vi "Set Switch State V2.vi"(5 "Action":T1(ring)=enum."Connect PulseGen to CH2", 7 "State":bool, 11 "error in (no error)":errorcluster) -> (15 "error out":errorcluster)   [LabVIEW 2010]
uses:
  <vilib>/DAQmx/write.llb/DAQmx Write (Digital 1D Bool 1Chan 1Samp).vi
  <vilib>/DAQmx/write.llb/DAQmx Write (Digital U8 1Chan 1Samp).vi
  <vilib>/DAQmx/create/channels.llb/DAQmx Create Channel (DO-Digital Output).vi
  <vilib>/daqmx/miscellaneous.llb/DAQmx Fill In Error Info.vi
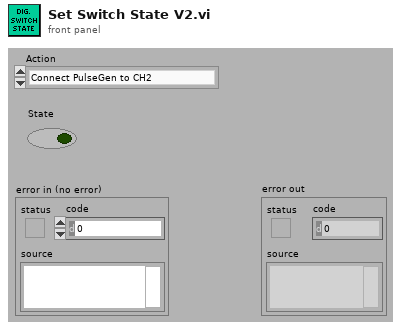
[diagram p1: front panel]
types:
  T1 = enum16{"--Disconnect All--", "Connect PulseGen to CH1", "Connect PulseGen to CH2", "Connect PulseGen to CH3", "Connect PulseGen to CH4", "Connect PulseGen to CH5", "Connect PulseGen to CH6", "Connect PulseGen to CH7", "Connect PulseGen to CH8", "Connect PulseGen to CH9", "Connect PulseGen to CH10", "Connect PulseGen to CH11", "Connect PulseGen to CH12", "Connect PulseGen to CH13", "Connect PulseGen to CH14", "Connect PulseGen to CH15", "Connect PulseGen to CH16", "Connect PulseGen to CH17", "Connect PulseGen to CH18", "Connect PulseGen to CH19", "Connect PulseGen to CH20", "Connect PulseGen to CH21", "Connect PulseGen to CH22", "Connect PulseGen to CH23", "Connect PulseGen to CH24", "Connect PulseGen to CH25", "Set MAG_SW", "Set Dynamic Load", "Set Expansion Trigger", "Trigger Positive Pulse", "Trigger Negative Pulse", "Set MSP Magic Pin", "Set BAT_EN", "Connect MSP_ACLK to CTR", "Connect MSP_MCLK to CTR", "Connect MSP_DIG_TST_OUT to CTR", "Connect STIM_SCK to CTR", "Connect STIM_CLK to CTR", "Connect SMU2 to Magnet", "Magnet Enable", "Cap Short", "Connect Positive Pulse to Pulse Bus", "Connect Negative Pulse to Pulse Bus", "Connect JTAG", "Connect JTAG DVDD Power", "RF Attach", "Connect SMU3 to VBAT", "Connect SMU3 Soft Start", "Connect ARB to Charge Coil", "Connect ARB to Matrix", "Connect CTR to Matrix", "DMM_I Short", "DMM_I 1000 Ohm", "DMM_I 100 Ohm", "DMM_I 10 Ohm", "Connect CH25 to DUT GND", "Enclosure Lights", "Heat Fan Zone 1", "Heat Fan Zone 2", "Temp Zone 1", "Temp Zone 2", "Temp Zone 3", "Guard Door Locks", "Air Heat Zone 3", "Zone 3 Vent", "Zone 3 Loader", "Zone 3 Upper Bed", "Zone 3 Lower Bed", "Zone 3 Standby Temp", "Yellow Light", "Red Light", "Green Light", "Reset Common Test Lines"}
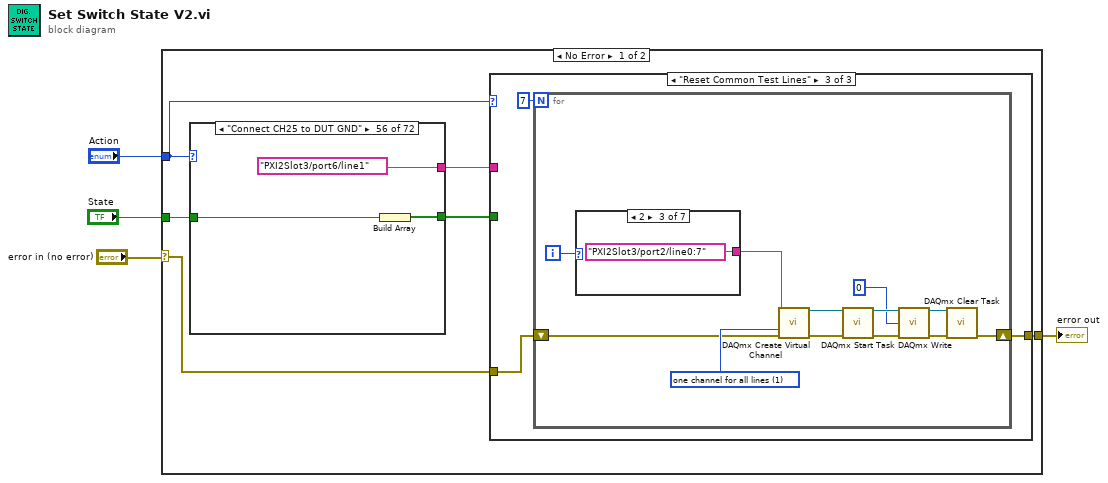
[diagram p0: block diagram]
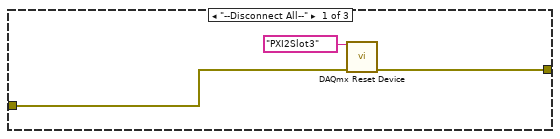
[diagram p2: hidden frame]
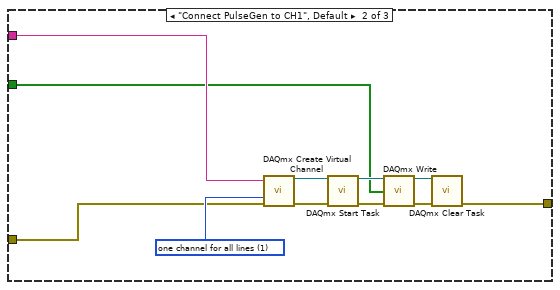
[diagram p3: hidden frame]
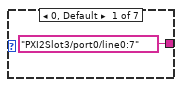
[diagram p4: hidden frame]
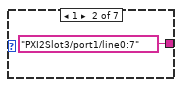
[diagram p5: hidden frame]
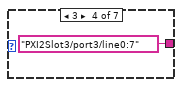
[diagram p6: hidden frame]
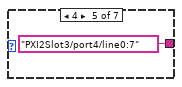
[diagram p7: hidden frame]
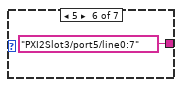
[diagram p8: hidden frame]
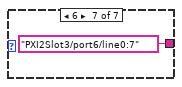
[diagram p9: hidden frame]
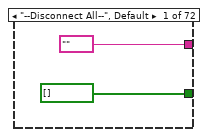
[diagram p10: hidden frame]
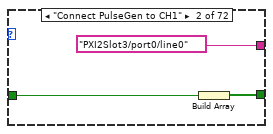
[diagram p11: hidden frame]
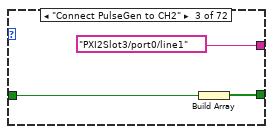
[diagram p12: hidden frame]
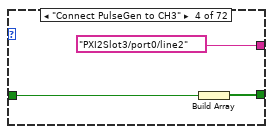
[diagram p13: hidden frame]
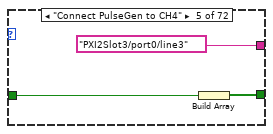
[diagram p14: hidden frame]
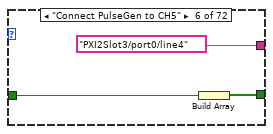
[diagram p15: hidden frame]
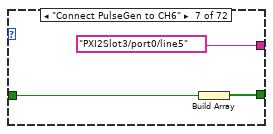
[diagram p16: hidden frame]
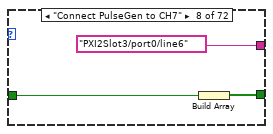
[diagram p17: hidden frame]
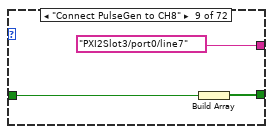
[diagram p18: hidden frame]
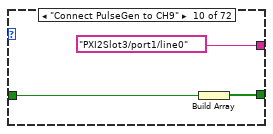
[diagram p19: hidden frame]
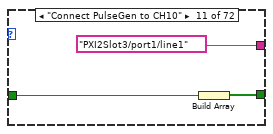
[diagram p20: hidden frame]
diagram:
  n1 = case shown="No Error" "error in (no error)" {
    selector: "error in (no error)" -> [w5 w263]
    tunnel: "State" -> [w8 _]
    tunnel: [w7 w263] -> w3
    tunnel: "Action" -> [w6 _]
    frame No Error {
      n2 = case shown="\"Connect CH25 to DUT GND\"" w6 {
        tunnel: [tag "" ("Lines") tag "PXI2Slot3/port0/line0" ("Lines") tag "PXI2Slot3/port0/line1" ("Lines") tag "PXI2Slot3/port0/line2" ("Lines") tag "PXI2Slot3/port0/line3" ("Lines") tag "PXI2Slot3/port0/line4" ("Lines") tag "PXI2Slot3/port0/line5" ("Lines") tag "PXI2Slot3/port0/line6" ("Lines") tag "PXI2Slot3/port0/line7" ("Lines") tag "PXI2Slot3/port1/line0" ("Lines") tag "PXI2Slot3/port1/line1" ("Lines") tag "PXI2Slot3/port1/line2" ("Lines") tag "PXI2Slot3/port1/line3" ("Lines") tag "PXI2Slot3/port1/line4" ("Lines") tag "PXI2Slot3/port1/line5" ("Lines") tag "PXI2Slot3/port1/line6" ("Lines") tag "PXI2Slot3/port1/line7" ("Lines") tag "PXI2Slot3/port2/line0" ("Lines") tag "PXI2Slot3/port2/line1" ("Lines") tag "PXI2Slot3/port2/line2" ("Lines") tag "PXI2Slot3/port2/line3" ("Lines") tag "PXI2Slot3/port2/line4" ("Lines") tag "PXI2Slot3/port2/line5" ("Lines") tag "PXI2Slot3/port2/line6" ("Lines") tag "PXI2Slot3/port2/line7" ("Lines") tag "PXI2Slot3/port3/line0" ("Lines") tag "PXI2Slot3/port3/line1" ("Lines") tag "PXI2Slot3/port3/line2:3" ("Lines") tag "PXI2Slot3/port3/line3" ("Lines") tag "PXI2Slot3/port3/line3:4" ("Lines") tag "PXI2Slot3/port3/line3:5" ("Lines") tag "PXI2Slot3/port3/line6" ("Lines") tag "PXI2Slot3/port3/line7" ("Lines") tag "PXI2Slot3/port4/line0" ("Lines") tag "PXI2Slot3/port4/line1" ("Lines") tag "PXI2Slot3/port4/line2" ("Lines") tag "PXI2Slot3/port4/line3" ("Lines") tag "PXI2Slot3/port4/line4" ("Lines") tag "PXI2Slot3/port4/line5" ("Lines") tag "PXI2Slot3/port4/line6" ("Lines") tag "PXI2Slot3/port4/line7" ("Lines") tag "PXI2Slot3/port5/line0" ("Lines") tag "PXI2Slot3/port5/line1" ("Lines") tag "PXI2Slot3/port5/line2" ("Lines") tag "PXI2Slot3/port5/line3" ("Lines") tag "PXI2Slot3/port5/line4" ("Lines") tag "PXI2Slot3/port5/line5" ("Lines") tag "PXI2Slot3/port5/line6" ("Lines") tag "PXI2Slot3/port5/line7" ("Lines") tag "PXI2Slot3/port6/line7" ("Lines") tag "PXI2Slot3/port6/line6" ("Lines") tag "PXI2Slot3/port6/line5" ("Lines") tag "PXI2Slot3/port6/line4" ("Lines") tag "PXI2Slot3/port6/line3" ("Lines") tag "PXI2Slot3/port6/line2" ("Lines") tag "PXI2Slot3/port6/line1" ("Lines") tag "PXI2Slot3/port8/line0" ("Lines") tag "PXI2Slot3/port8/line1" ("Lines") tag "PXI2Slot3/port8/line2" ("Lines") tag "PXI2Slot3/port8/line3" ("Lines") tag "PXI2Slot3/port8/line4" ("Lines") tag "PXI2Slot3/port8/line5" ("Lines") tag "PXI2Slot3/port8/line6" ("Lines") tag "PXI2Slot3/port8/line7" ("Lines") tag "PXI2Slot3/port9/line0" ("Lines") tag "PXI2Slot3/port9/line1" ("Lines") tag "PXI2Slot3/port9/line2" ("Lines") tag "PXI2Slot3/port9/line3" ("Lines") tag "PXI2Slot3/port9/line4" ("Lines") tag "PXI2Slot3/port9/line5" ("Lines") tag "PXI2Slot3/port9/line6" ("Lines") tag "PXI2Slot3/port9/line7" ("Lines")] -> w10
        tunnel: [bool[] [] w50 w53 w56 w59 w62 w65 w68 w71 w74 w77 w80 w83 w86 w89 w92 w95 w98 w101 w104 w107 w110 w113 w116 w119 w122 w125 w128 w131 w134 w138 w141 w144 w147 w150 w153 w156 w159 w162 w165 w168 w171 w174 w177 w180 w183 w186 w189 w192 w195 w198 w201 w204 w207 w210 w213 w216 w219 w222 w226 w229 w231 w234 w237 w240 w244 w246 w249 w252 w255 w258 w261] -> w9
        tunnel: w8 -> [_ w49 w52 w55 w58 w61 w64 w67 w70 w73 w76 w79 w82 w85 w88 w91 w94 w97 w100 w103 w106 w109 w112 w115 w118 w121 w124 w127 w130 w133 w137 w140 w143 w146 w149 w152 w155 w158 w161 w164 w167 w170 w173 w176 w179 w182 w185 w188 w191 w194 w197 w200 w203 w206 w209 w212 w215 w218 w221 w225 w228 w230 w233 w236 w239 w243 w245 w248 w251 w254 w257 w260]
        frame "--Disconnect All--", Default {
        }
        frame "Connect PulseGen to CH1" {
          n3 = Build Array(w49) -> (w50:bool[])
        }
        frame "Connect PulseGen to CH2" {
          n4 = Build Array(w52) -> (w53:bool[])
        }
        frame "Connect PulseGen to CH3" {
          n5 = Build Array(w55) -> (w56:bool[])
        }
        frame "Connect PulseGen to CH4" {
          n6 = Build Array(w58) -> (w59:bool[])
        }
        frame "Connect PulseGen to CH5" {
          n7 = Build Array(w61) -> (w62:bool[])
        }
        frame "Connect PulseGen to CH6" {
          n8 = Build Array(w64) -> (w65:bool[])
        }
        frame "Connect PulseGen to CH7" {
          n9 = Build Array(w67) -> (w68:bool[])
        }
        frame "Connect PulseGen to CH8" {
          n10 = Build Array(w70) -> (w71:bool[])
        }
        frame "Connect PulseGen to CH9" {
          n11 = Build Array(w73) -> (w74:bool[])
        }
        frame "Connect PulseGen to CH10" {
          n12 = Build Array(w76) -> (w77:bool[])
        }
        frame "Connect PulseGen to CH11" {
          n13 = Build Array(w79) -> (w80:bool[])
        }
        frame "Connect PulseGen to CH12" {
          n14 = Build Array(w82) -> (w83:bool[])
        }
        frame "Connect PulseGen to CH13" {
          n15 = Build Array(w85) -> (w86:bool[])
        }
        frame "Connect PulseGen to CH14" {
          n16 = Build Array(w88) -> (w89:bool[])
        }
        frame "Connect PulseGen to CH15" {
          n17 = Build Array(w91) -> (w92:bool[])
        }
        frame "Connect PulseGen to CH16" {
          n18 = Build Array(w94) -> (w95:bool[])
        }
        frame "Connect PulseGen to CH17" {
          n19 = Build Array(w97) -> (w98:bool[])
        }
        frame "Connect PulseGen to CH18" {
          n20 = Build Array(w100) -> (w101:bool[])
        }
        frame "Connect PulseGen to CH19" {
          n21 = Build Array(w103) -> (w104:bool[])
        }
        frame "Connect PulseGen to CH20" {
          n22 = Build Array(w106) -> (w107:bool[])
        }
        frame "Connect PulseGen to CH21" {
          n23 = Build Array(w109) -> (w110:bool[])
        }
        frame "Connect PulseGen to CH22" {
          n24 = Build Array(w112) -> (w113:bool[])
        }
        frame "Connect PulseGen to CH23" {
          n25 = Build Array(w115) -> (w116:bool[])
        }
        frame "Connect PulseGen to CH24" {
          n26 = Build Array(w118) -> (w119:bool[])
        }
        frame "Connect PulseGen to CH25" {
          n27 = Build Array(w121) -> (w122:bool[])
        }
        frame "Set MAG_SW" {
          n28 = Build Array(w124) -> (w125:bool[])
        }
        frame "Set Dynamic Load" {
          n29 = Build Array(w127, w127) -> (w128:bool[])
        }
        frame "Set Expansion Trigger" {
          n30 = Build Array(w130) -> (w131:bool[])
        }
        frame "Trigger Positive Pulse" {
          n31 = Build Array(w133, w133) -> (w134:bool[])
        }
        frame "Trigger Negative Pulse" {
          n32 = Build Array(w137, FALSE ("element"), w137) -> (w138:bool[])
        }
        frame "Set MSP Magic Pin" {
          n33 = Build Array(w140) -> (w141:bool[])
        }
        frame "Set BAT_EN" {
          n34 = Build Array(w143) -> (w144:bool[])
        }
        frame "Connect MSP_ACLK to CTR" {
          n35 = Build Array(w146) -> (w147:bool[])
        }
        frame "Connect MSP_MCLK to CTR" {
          n36 = Build Array(w149) -> (w150:bool[])
        }
        frame "Connect MSP_DIG_TST_OUT to CTR" {
          n37 = Build Array(w152) -> (w153:bool[])
        }
        frame "Connect STIM_SCK to CTR" {
          n38 = Build Array(w155) -> (w156:bool[])
        }
        frame "Connect STIM_CLK to CTR" {
          n39 = Build Array(w158) -> (w159:bool[])
        }
        frame "Connect SMU2 to Magnet" {
          n40 = Build Array(w161) -> (w162:bool[])
        }
        frame "Magnet Enable" {
          n41 = Build Array(w164) -> (w165:bool[])
        }
        frame "Cap Short" {
          n42 = Build Array(w167) -> (w168:bool[])
        }
        frame "Connect Positive Pulse to Pulse Bus" {
          n43 = Build Array(w170) -> (w171:bool[])
        }
        frame "Connect Negative Pulse to Pulse Bus" {
          n44 = Build Array(w173) -> (w174:bool[])
        }
        frame "Connect JTAG" {
          n45 = Build Array(w176) -> (w177:bool[])
        }
        frame "Connect JTAG DVDD Power" {
          n46 = Build Array(w179) -> (w180:bool[])
        }
        frame "RF Attach" {
          n47 = Build Array(w182) -> (w183:bool[])
        }
        frame "Connect SMU3 to VBAT" {
          n48 = Build Array(w185) -> (w186:bool[])
        }
        frame "Connect SMU3 Soft Start" {
          n49 = Build Array(w188) -> (w189:bool[])
        }
        frame "Connect ARB to Charge Coil" {
          n50 = Build Array(w191) -> (w192:bool[])
        }
        frame "Connect ARB to Matrix" {
          n51 = Build Array(w194) -> (w195:bool[])
        }
        frame "Connect CTR to Matrix" {
          n52 = Build Array(w197) -> (w198:bool[])
        }
        frame "DMM_I Short" {
          n53 = Build Array(w200) -> (w201:bool[])
        }
        frame "DMM_I 1000 Ohm" {
          n54 = Build Array(w203) -> (w204:bool[])
        }
        frame "DMM_I 100 Ohm" {
          n55 = Build Array(w206) -> (w207:bool[])
        }
        frame "DMM_I 10 Ohm" {
          n56 = Build Array(w209) -> (w210:bool[])
        }
        frame "Connect CH25 to DUT GND" {
          n57 = Build Array(w212) -> (w213:bool[])
        }
        frame "Enclosure Lights" {
          n58 = Build Array(w215) -> (w216:bool[])
        }
        frame "Heat Fan Zone 1" {
          n59 = Build Array(w218) -> (w219:bool[])
        }
        frame "Heat Fan Zone 2" {
          n60 = Build Array(w221) -> (w222:bool[])
        }
        frame "Temp Zone 1" {
          n61 = Build Array(w225) -> (w226:bool[])
        }
        frame "Temp Zone 2" {
          n62 = Build Array(w228) -> (w229:bool[])
        }
        frame "Temp Zone 3" {
          n63 = Build Array(w230) -> (w231:bool[])
        }
        frame "Guard Door Locks" {
          n64 = Build Array(w233) -> (w234:bool[])
        }
        frame "Air Heat Zone 3" {
          n65 = Build Array(w236) -> (w237:bool[])
        }
        frame "Zone 3 Vent" {
          n66 = Build Array(w239) -> (w240:bool[])
        }
        frame "Zone 3 Loader" {
          n67 = Build Array(w243) -> (w244:bool[])
        }
        frame "Zone 3 Upper Bed" {
          n68 = Build Array(w245) -> (w246:bool[])
        }
        frame "Zone 3 Lower Bed" {
          n69 = Build Array(w248) -> (w249:bool[])
        }
        frame "Zone 3 Standby Temp" {
          n70 = Build Array(w251) -> (w252:bool[])
        }
        frame "Yellow Light" {
          n71 = Build Array(w254) -> (w255:bool[])
        }
        frame "Red Light" {
          n72 = Build Array(w257) -> (w258:bool[])
        }
        frame "Green Light" {
          n73 = Build Array(w260) -> (w261:bool[])
        }
      }
      n74 = case shown="\"Reset Common Test Lines\"" w6 {
        tunnel: w10 -> [_ w17 _]
        tunnel: w9 -> [_ w16 _]
        tunnel: [w13 w15 w27] -> w7
        tunnel: w5 -> [w11 w14 w25]
        frame "--Disconnect All--" {
          n75 = call <vilib>:"DAQmx Reset Device.vi"("device in"=tag "PXI2Slot3", "error in"=w11) -> ("error out"=w13:errorcluster)  [unwired: 13 in]
        }
        frame "Connect PulseGen to CH1", Default {
          w22 = 1 items=["one channel for each line", "one channel for all lines"] ("line grouping")
          n76 = call-poly <vilib>:"DAQmx Create Virtual Channel.vi"("lines"=w17, "line grouping"=w22, "error in"=w14) -> ("task out"=w24:refnum<k21>, "error out"=w23:errorcluster)  [unwired: 11 in]
          n77 = call <vilib>:"DAQmx Start Task.vi"("task/channels in"=w24, "error in"=w23) -> ("task out"=w21:refnum<k21>, "error out"=w20:errorcluster)  [unwired: 12 in]
          n78 = call-poly <vilib>:"DAQmx Write.vi"("task/channels in"=w21, "data"=w16, "error in"=w20) -> ("task out"=w19:refnum<k21>, "error out"=w18:errorcluster)  [unwired: 10 in, 1 out]
          n79 = call <vilib>:"DAQmx Clear Task.vi"("task in"=w19, "error in"=w18) -> ("error out"=w15:errorcluster)  [unwired: 13 in]
        }
        frame "Reset Common Test Lines" {
          n80 = for {
            N: 7 -> [_]
            shift-right: [w32] -> w27
            shift-left: w25 -> [w30]
            i -> [w28]
            w37 = 1 items=["one channel for each line", "one channel for all lines"] ("line grouping")
            n81 = case shown="2" w28 {
              tunnel: [tag "PXI2Slot3/port0/line0:7" ("lines") tag "PXI2Slot3/port1/line0:7" ("lines") tag "PXI2Slot3/port2/line0:7" ("lines") tag "PXI2Slot3/port3/line0:7" ("lines") tag "PXI2Slot3/port4/line0:7" ("lines") tag "PXI2Slot3/port5/line0:7" ("lines") tag "PXI2Slot3/port6/line0:7" ("lines")] -> w29
              frame 0, Default {
              }
              frame 1 {
              }
              frame 2 {
              }
              frame 3 {
              }
              frame 4 {
              }
              frame 5 {
              }
              frame 6 {
              }
            }
            n82 = call-poly <vilib>:"DAQmx Create Virtual Channel.vi"("lines"=w29, "line grouping"=w37, "error in"=w30) -> ("task out"=w39:refnum<k21>, "error out"=w38:errorcluster)  [unwired: 11 in]
            n83 = call <vilib>:"DAQmx Start Task.vi"("task/channels in"=w39, "error in"=w38) -> ("task out"=w36:refnum<k21>, "error out"=w35:errorcluster)  [unwired: 12 in]
            n84 = call-poly <vilib>:"DAQmx Write.vi"("task/channels in"=w36, "data"=u8 0, "error in"=w35) -> ("task out"=w34:refnum<k21>, "error out"=w33:errorcluster)  [unwired: 10 in, 1 out]
            n85 = call <vilib>:"DAQmx Clear Task.vi"("task in"=w34, "error in"=w33) -> ("error out"=w32:errorcluster)  [unwired: 13 in]
          }
        }
      }
    }
    frame Error {
    }
  }
  "error out" <- w3
